vi "SendPrintLine.vi"(8 "error in (no error)":errorcluster, 9 "Color":u32(colorbox), 10 "e":string, 11 "DownStreamMsgHandler in":refnum<class "DownStreamMsgHandler.lvclass">) -> (0 "error out":errorcluster, 3 "DownStreamMsgHandler out":refnum<class "DownStreamMsgHandler.lvclass">)   [LabVIEW 2020, in "DownstreamMsgHandler.lvlib" / "DownStreamMsgHandler.lvclass"]
uses:
  DownStreamMsgHandler.lvclass
  UpstreamMsg/PrintF/Msg.ctl
  UpstreamMsg/PrintF/PrintF.lvclass
  C:/Users/taylo/Projects/g-go-service-fwrk/scratchpad/ServiceManagerBeta/ServiceManager/UpstreamMsg/UpstreamMsgParent/UpstreamMsgParent.lvclass
  C:/Users/taylo/Projects/g-go-service-fwrk/scratchpad/ServiceManagerBeta/ServiceManager/UpstreamMsg/PrintF/PrintF.lvclass
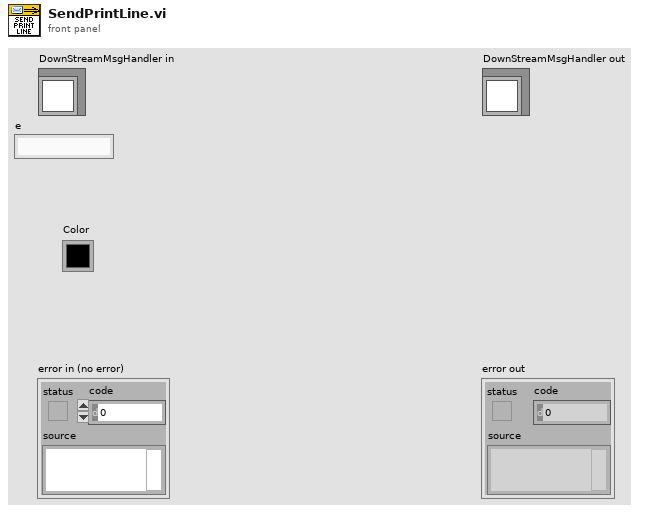
[diagram p1: front panel]
types:
  T1 = typedef "UpstreamMsg.lvlib/PrintF.lvclass/Msg.ctl" = cluster{"TxtColor":cluster{"r":u8, "b":u8, "g":u8}, "LineToPrint":string}
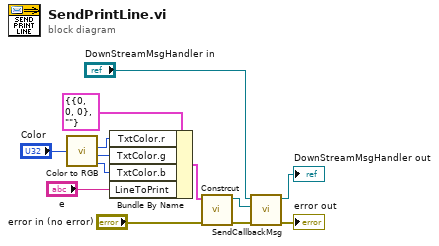
[diagram p0: block diagram]
diagram:
  n1 = call <vilib>:"Color to RGB.vi"("Color"="Color") -> ("R"=w5:u8, "G"=w4:u8, "B"=w1:u8)  [unwired: 1 out]
  n2 = Bundle By Name(cluster=T1 {"TxtColor"={"r"=0, "b"=0, "g"=0}, "LineToPrint"=""} ("PrintLine"), "TxtColor.r"=w5, "TxtColor.g"=w4, "TxtColor.b"=w1, "LineToPrint"="e") -> (w6:T1)
  n3 = call "Constrcut.vi"("error in (no error)"="error in (no error)", "PrintLine"=w6) -> ("error out"=w11:errorcluster, "PrintF out"=w12:refnum<class "PrintF.lvclass">)  [unwired: 8 in]
  n4 = call-dynamic "SendCallbackMsg.vi"("error in (no error)"=w11, "UpstreamMsg"=w12, "DownStreamMsgHandler in"="DownStreamMsgHandler in") -> ("error out"=→"error out":errorcluster, "DownStreamMsgHandler out"=→"DownStreamMsgHandler out":refnum<class "DownStreamMsgHandler.lvclass">)  [unwired: 7 in]
